vi "LNOPA01 Utility Parse Function From String.vi .vi"(8 "error in (no error)":errorcluster, 9 "Function String":string, 11 "VISA session":refnum<visa-resource-name>) -> (0 "error out":errorcluster, 1 "Modifier":i32[](array[ring]) items=["None", "Minimum", "Maximum", "Integral Positive", "Integral Negative", "Integral"], 2 "Measurement":i32[](array[ring]) items=["Voltage True RMS", "Voltage Mean", "Voltage Rectified Mean ", "Voltage Peak-To-Peak ", "Voltage Highest Value ", "Voltage Lowest Value ", "Voltage Crest Factor", "Voltage Absolute Phase", "Voltage True RMS Phase-To-Phase", "Voltage Harmonic", "Voltage TRMS Phase-To-Phase Harmonic", "Voltage Form Factor", "Voltage Harmonic Content", "Voltage Fundamental Content", "Voltage THD", "Current True RMS", "Current Mean", "Current Rectified Mean ", "Current Peak-To-Peak ", "Current Highest Value ", "Current Lowest Value", "Current Crest Factor", "Current Absolute Phase", "Current Harmonic", "Current Form Factor", "Current Harmonic Content", "Current Fundamental Content", "Current THD", "Power Active", "Power Apparent", "Power Reactive", "Power Factor", "Power Active Harmonic", "Power Apparent Harmonic", "Power Reactive Harmonic", "Power Factor Harmonic", "Power Corrected", "Phase", "Phase Harmonic", "Impedance", "Resistance Serial", "Resistance Parallel", "Reactance Serial", "Reactance Parallel", "Impedance Harmonic", "Resistance Serial Harmonic", "Resistance Parallel Harmonic", "Reactance Serial Harmonic", "Reactance Parallel Harmonic", "Frequency", "Averaging Interval", "Shaft Torque", "Rotational Speed", "Mechanical Power", "Rotational Asynchronousity", "Motor Efficiency", "Raw Process Input Value ", "Voltage Mean Phase-To-Phase", "Voltage Rectified Mean Phase-To-Phase", "Voltage Form Factor Phase-To-Phase", "Averaging Interval Relative Timestamp", "Electrical Efficiency", "Electrical Efficiency Harmonic", "True RMS Voltage Without DC", "True RMS Current Without DC"], 3 "dup VISA session":refnum<visa-resource-name>, 4 "Phase":i32[](array[numeric]) min=-1 max=64 step=1)   [LabVIEW 2009]
doc: "This VI parses the function string returned from the instrument to the arrays."
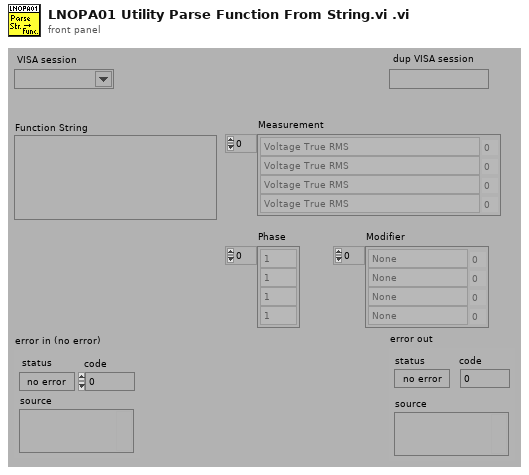
[diagram p1: front panel]
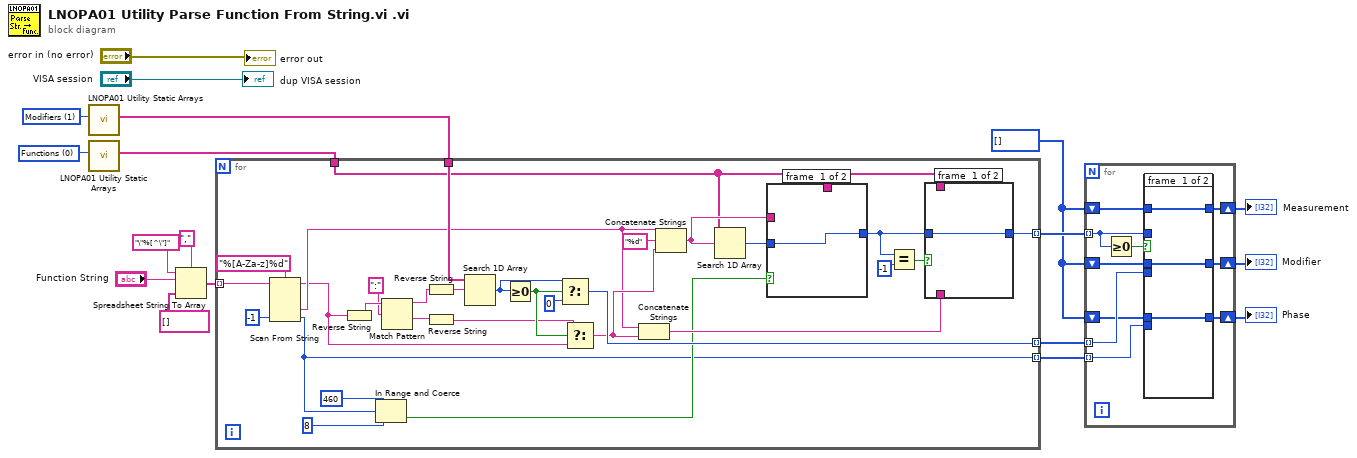
[diagram p0: block diagram]
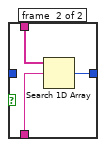
[diagram p2: hidden frame]
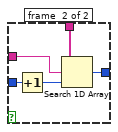
[diagram p3: hidden frame]
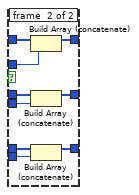
[diagram p4: hidden frame]
diagram:
  w8 = u16 0 items=["Functions", "Modifiers"] ("Array")
  w10 = u16 1 items=["Functions", "Modifiers"] ("Array")
  w12 = i32[] [] ("Array Constant")
  n1 = call "LNOPA01 Utility Static Arrays.vi"("Array"=w10) -> ("Array Out"=w11:string[])  [unwired: 9 in, 1 out]
  n2 = call "LNOPA01 Utility Static Arrays.vi"("Array"=w8) -> ("Array Out"=w9:string[])  [unwired: 9 in, 1 out]
  n3 = Spreadsheet String To Array(delimiter (Tab)=",", format string="\"%[^\"]", spreadsheet string="Function String", array type (2D Dbl)=string[] [] ("Array Constant")) -> (array=w6:string[])
  n4 = for {
    tunnel: w6 -> [w46] mode=indexing
    tunnel: [w47] -> w15 mode=indexing
    tunnel: w11 -> [w48]
    tunnel: w9 -> [w38]
    tunnel: [w19] -> w16 mode=indexing
    tunnel: [w33] -> w13 mode=indexing
    n5 = Scan From String(format string="%[A-Za-z]%d" ("Format String"), input string=w46, default 2=-1 ("Default Value 2")) -> (remaining string=w23:string, output 1=w35:string, output 2=w19:i32)  [unwired: 3 in, 2 out]
    n6 = Reverse String(1:w23) -> (0:w31:string)
    n7 = In Range and Coerce(upper limit=460 ("y"), x=w19, lower limit=8 ("y")) -> (In Range?=w20:bool)  [unwired: 1 out]
    n8 = Match Pattern(string=w31, regular expression=":" ("search char (-)")) -> (before substring=w29:string, after substring=w27:string)  [unwired: 1 in, 2 out]
    n9 = Reverse String(1:w29) -> (0:w28:string)
    n10 = Reverse String(1:w27) -> (0:w24:string)
    n11 = Search 1D Array(1D array=w48, element=w28) -> (index of element=w25:i32)  [unwired: 1 in]
    n12 = Greater Or Equal To 0?(x=w25) -> (x >= 0?=w43:bool)
    n13 = Select(t=w25, s=w43, f=0 ("t")) -> (s? t:f=w47:i32)
    n14 = Select(t=w24, s=w43, f=w23) -> (s? t:f=w36:string)
    n15 = Concatenate Strings(w35, w36) -> (w34:string)
    n16 = Concatenate Strings(w35, "%d" ("Substring"), w36) -> (w41:string)
    n17 = Search 1D Array(1D array=w38, element=w41) -> (index of element=w42:i32)  [unwired: 1 in]
    n18 = case shown="True" w20 {
      tunnel: w42 -> [w53 w58]
      tunnel: [w53 w55] -> w32
      tunnel: w38 -> [_ w57]
      tunnel: w41 -> [_ w56]
      frame #0 {
      }
      frame #1 {
        n19 = Increment(x=w58) -> (x+1=w54:i32)
        n20 = Search 1D Array(1D array=w57, element=w56, start index (0)=w54) -> (index of element=w55:i32)
      }
    }
    n21 = Equal?(x=w32, y=-1) -> (x = y?=w37:bool)
    n22 = case shown="True" w37 {
      tunnel: w38 -> [_ w52]
      tunnel: w34 -> [_ w51]
      tunnel: [w49 w50] -> w33
      tunnel: w32 -> [w49 _]
      frame #0 {
      }
      frame #1 {
        n23 = Search 1D Array(1D array=w52, element=w51) -> (index of element=w50:i32)  [unwired: 1 in]
      }
    }
  }
  n24 = for {
    shift-right: [w67] -> w14
    shift-left: w12 -> [w68]
    shift-right: [w62] -> w17
    shift-left: w12 -> [w64]
    shift-right: [w59] -> w18
    shift-left: w12 -> [w61]
    tunnel: w13 -> [w65] mode=indexing
    tunnel: w15 -> [w63] mode=indexing
    tunnel: w16 -> [w60] mode=indexing
    n25 = Greater Or Equal To 0?(x=w65) -> (x >= 0?=w66:bool)
    n26 = case shown="False" w66 {
      tunnel: w68 -> [w71 w80]
      tunnel: w65 -> [_ w79]
      tunnel: [w71 w78] -> w67
      tunnel: w64 -> [w70 w77]
      tunnel: w63 -> [_ w76]
      tunnel: [w70 w75] -> w62
      tunnel: w61 -> [w69 w74]
      tunnel: w60 -> [_ w73]
      tunnel: [w69 w72] -> w59
      frame #0 {
      }
      frame #1 {
        n27 = Build Array (concatenate)(w80, w79) -> (w78:i32[])
        n28 = Build Array (concatenate)(w77, w76) -> (w75:i32[])
        n29 = Build Array (concatenate)(w74, w73) -> (w72:i32[])
      }
    }
  }
  "Measurement" <- w14
  "Phase" <- w18
  "Modifier" <- w17
  "error out" <- "error in (no error)"
  "dup VISA session" <- "VISA session"
